vi "DB Tools Fetch Element Data.vi"   [LabVIEW 2020, in "NI_Database_API.lvlib"]
doc: "Retrieves the data located at the <B>column index</B> of the current record in the recordset identified by the <B>recordset reference</B>. The <B>column index</B> can be either the zero-indexed position of the column in the recordset or the name of the column. Wire data to the <B>type</B> input to determine the polymorphic instance to use or manually select the instance."
uses:
  <vilib>/addons/database/NI_Database_API.lvlib
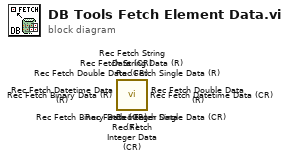
[diagram p0: block diagram]
diagram:
  n1 = call <vilib>:"Rec Fetch Integer Data (R).vi"() -> ()  [unwired: 7 in, 3 out]
  n2 = call <vilib>:"Rec Fetch Single Data (R).vi"() -> ()  [unwired: 7 in, 3 out]
  n3 = call <vilib>:"Rec Fetch Datetime Data (R).vi"() -> ()  [unwired: 7 in, 3 out]
  n4 = call <vilib>:"Rec Fetch Double Data (R).vi"() -> ()  [unwired: 7 in, 3 out]
  n5 = call <vilib>:"Rec Fetch String Data (R).vi"() -> ()  [unwired: 7 in, 3 out]
  n6 = call <vilib>:"Rec Fetch Double Data (CR).vi"() -> ()  [unwired: 7 in, 3 out]
  n7 = call <vilib>:"Rec Fetch Integer Data (CR).vi"() -> ()  [unwired: 7 in, 3 out]
  n8 = call <vilib>:"Rec Fetch Single Data (CR).vi"() -> ()  [unwired: 7 in, 3 out]
  n9 = call <vilib>:"Rec Fetch String Data (CR).vi"() -> ()  [unwired: 7 in, 3 out]
  n10 = call <vilib>:"Rec Fetch Datetime Data (CR).vi"() -> ()  [unwired: 7 in, 3 out]
  n11 = call <vilib>:"Rec Fetch Binary Data (CR).vi"() -> ()  [unwired: 7 in, 3 out]
  n12 = call <vilib>:"Rec Fetch Binary Data (R).vi"() -> ()  [unwired: 7 in, 3 out]
